vi "ControlDriveDistance.vi"(11 "Robot Motion Commands":T1) -> ()   [LabVIEW 2018]
uses:
  Controls/Robot Pivot Motion Commands.ctl
  Controls/Pivot Motor Commands.ctl
  Controls/Robot Drive Mode.ctl
  <vilib>/Rock Robotics/WPI/Utilities/WPI_GetSetVariantRefNum.vi
  <vilib>/addons/control/pid/pid.llb/PID (DBL Array).vi
  <vilib>/addons/control/pid/NI_PID_pid.lvlib
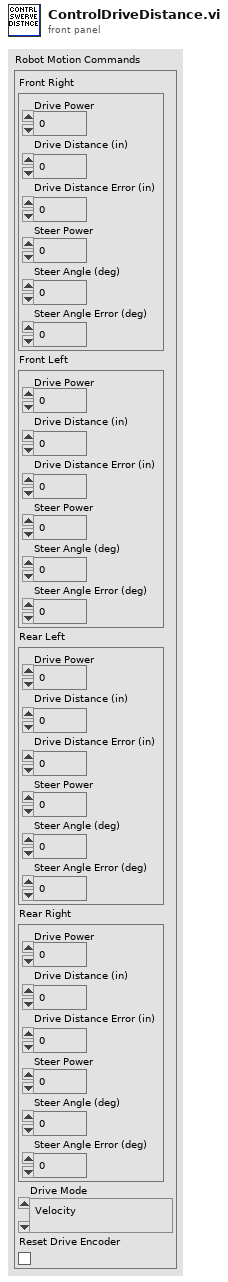
[diagram p1: front panel]
types:
  T1 = typedef "Robot Pivot Motion Commands.ctl" = cluster{"Front Right":T2, "Front Left":T2, "Rear Left":T2, "Rear Right":T2, "Drive Mode":T3, "Reset Drive Encoder":bool}
  T2 = typedef "Pivot Motor Commands.ctl" = cluster{"Drive Power":dbl, "Drive Distance (in)":dbl, "Drive Distance Error (in)":dbl, "Steer Power":dbl, "Steer Angle (deg)":dbl, "Steer Angle Error (deg)":dbl}
  T3 = typedef "Robot Drive Mode.ctl" = enum16{"Velocity", "Distance"}
  T4 = cluster{"proportional gain (Kc)":dbl, "integral time (Ti, min)":dbl, "derivative time (Td, min)":dbl}
  T5 = cluster{"proportional gain (Kc)":dbl, "integral time (Ti, min)":dbl, "derivative time (Td, min)":dbl}[]
  T6 = typedef "WPI_RobotDriveDevRef.ctl" = cluster{"DevStatus":errorcluster, "Motors[]":T7[], "Square Inputs":bool, "Max Output":dbl}
  T7 = typedef "WPI_MotorControlDeviceRef.ctl" = cluster{"DeviceStatus":errorcluster, "Type":T8, "PWM":cluster{"PWM Channel":T9, "DeadBand":T10}, "CAN":cluster{"Device Number":u8, "SetOutput VI Ref":variant, "GetOutput VI Ref":variant, "Enable VI Ref":variant, "Disable VI Ref":variant, "Data":variant}, "Invert":bool, "DIO PWM":cluster{"PWM \"Enable\" Channel":T9, "DIOChannel":T11, "PWM Rate":dbl}}
  T8 = typedef "WPI_MotorControlType.ctl" = enum16{"PWM", "CAN", "DIO PWM"}
  T9 = typedef "FPGA_DIOPWMChannel.ctl" = enum8{"PWM 0", "PWM 1", "PWM 2", "PWM 3", "PWM 4", "PWM 5", "PWM 6", "PWM 7", "PWM 8", "PWM 9", "PWM MXP 0", "PWM MXP 1", "PWM MXP 2", "PWM MXP 3", "PWM MXP 4", "PWM MXP 5", "PWM MXP 6", "PWM MXP 7", "PWM MXP 8", "PWM MXP 9", "Invalid"}
  T10 = typedef "WPI_PWMDeadband.ctl" = cluster{"Name":string, "maxPositivePwm":i32, "minPositivePwm":i32, "centerPwm":i32, "maxNegativePwm":i32, "minNegativePwm":i32, "angularRange":u16}
  T11 = typedef "FPGA_DIOChannel.ctl" = enum8{"DIO 0", "DIO 1", "DIO 2", "DIO 3", "DIO 4", "DIO 5", "DIO 6", "DIO 7", "DIO 8", "DIO 9", "DIO MXP 0", "DIO MXP 1", "DIO MXP 2", "DIO MXP 3", "DIO MXP 4", "DIO MXP 5", "DIO MXP 6", "DIO MXP 7", "DIO MXP 8", "DIO MXP 9", "DIO MXP 10", "DIO MXP 11", "DIO MXP 12", "DIO MXP 13", "DIO MXP 14", "DIO MXP 15", "SPI Port CS1", "SPI Port CS2", "SPI Port CS3", "SPI Port MISO", "SPI Port MOSI", "Invalid"}
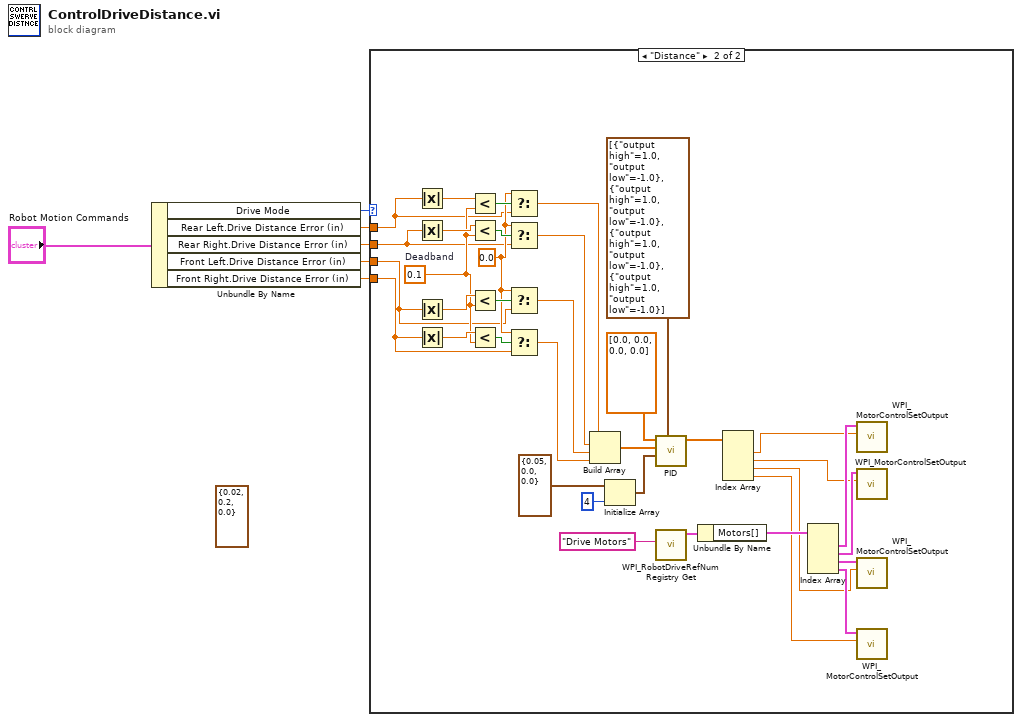
[diagram p0: block diagram]
diagram:
  (unwired) T4 {"proportional gain (Kc)"=0.02, "integral time (Ti, min)"=0.2, "derivative time (Td, min)"=0.0} ("PID gains")
  n1 = Unbundle By Name("Robot Motion Commands") -> ("Drive Mode"=w1:T3, "Rear Left.Drive Distance Error (in)"=w5:dbl, "Rear Right.Drive Distance Error (in)"=w4:dbl, "Front Left.Drive Distance Error (in)"=w2:dbl, "Front Right.Drive Distance Error (in)"=w3:dbl)
  n2 = case shown="\"Distance\"" w1 {
    tunnel: w5 -> [_ w10]
    tunnel: w4 -> [_ w9]
    tunnel: w3 -> [_ w8]
    tunnel: w2 -> [_ w7]
    frame "Velocity", Default {
      # "do nothing in velocity mode"
    }
    frame "Distance" {
      w16 = 0.0
      w11 = 0.1  # Deadband
      n3 = Absolute Value(x=w10) -> (abs(x)=w18:dbl)
      n4 = Absolute Value(x=w9) -> (abs(x)=w20:dbl)
      n5 = Absolute Value(x=w7) -> (abs(x)=w22:dbl)
      n6 = Absolute Value(x=w8) -> (abs(x)=w24:dbl)
      n7 = Less?(x=w18, y=w11) -> (x < y?=w17:bool)
      n8 = Less?(x=w20, y=w11) -> (x < y?=w19:bool)
      n9 = Less?(x=w22, y=w11) -> (x < y?=w21:bool)
      n10 = Less?(x=w24, y=w11) -> (x < y?=w23:bool)
      n11 = Select(t=w16, s=w17, f=w10) -> (s? t:f=w15:dbl)
      n12 = Select(t=w16, s=w19, f=w9) -> (s? t:f=w14:dbl)
      n13 = Select(t=w16, s=w21, f=w7) -> (s? t:f=w13:dbl)
      n14 = Select(t=w16, s=w23, f=w8) -> (s? t:f=w12:dbl)
      n15 = Build Array(w15, w14, w13, w12) -> (w35:dbl[])
      n16 = Initialize Array(T4 {"proportional gain (Kc)"=0.05, "integral time (Ti, min)"=0.0, "derivative time (Td, min)"=0.0} ("PID gains"), 4 ("dimension size")) -> (w36:T5)
      n17 = call-poly <vilib>:"PID.vi"("output range"=cluster{"output high":dbl, "output low":dbl}[] [{"output high"=1.0, "output low"=-1.0}, {"output high"=1.0, "output low"=-1.0}, {"output high"=1.0, "output low"=-1.0}, {"output high"=1.0, "output low"=-1.0}], "PID gains"=w36, "process variable"=w35, "setpoint"=dbl[] [0.0, 0.0, 0.0, 0.0]) -> ("output"=w33:dbl[])  [unwired: 6 in, 1 out]
      n18 = call <vilib>:"WPI_RobotDriveRefNum Registry Get.vi"("refnum name"="Drive Motors") -> ("RobotDriveDevRef"=w41:T6)  [unwired: 9 in, 1 out]
      n19 = Unbundle By Name(w41) -> ("Motors[]"=w34:T7[])
      n20 = Index Array(array=w33) -> (element #1=w28:dbl, element #2=w27:dbl, element #3=w26:dbl, element #4=w25:dbl)  [unwired: 4 in]
      n21 = Index Array(array=w34) -> (element #1=w32:T7, element #2=w31:T7, element #3=w30:T7, element #4=w29:T7)  [unwired: 4 in]
      n22 = call <vilib>:"WPI_MotorControlSetOutput.vi"("Output"=w28, "MotorControlDevRef"=w32) -> ()  [unwired: 7 in, 3 out]
      n23 = call <vilib>:"WPI_MotorControlSetOutput.vi"("Output"=w27, "MotorControlDevRef"=w31) -> ()  [unwired: 7 in, 3 out]
      n24 = call <vilib>:"WPI_MotorControlSetOutput.vi"("Output"=w26, "MotorControlDevRef"=w30) -> ()  [unwired: 7 in, 3 out]
      n25 = call <vilib>:"WPI_MotorControlSetOutput.vi"("Output"=w25, "MotorControlDevRef"=w29) -> ()  [unwired: 7 in, 3 out]
    }
  }
